vi "Normalize.vi"(11 "Data":dbl[][](array[numeric])) -> (0 "sx_all":dbl[][](array[numeric]), 2 "sx":dbl[](array[numeric]), 3 "Data_out":dbl[][](array[numeric]))   [LabVIEW 2014]
uses:
  <vilib>/Analysis/NI_AALBase.lvlib
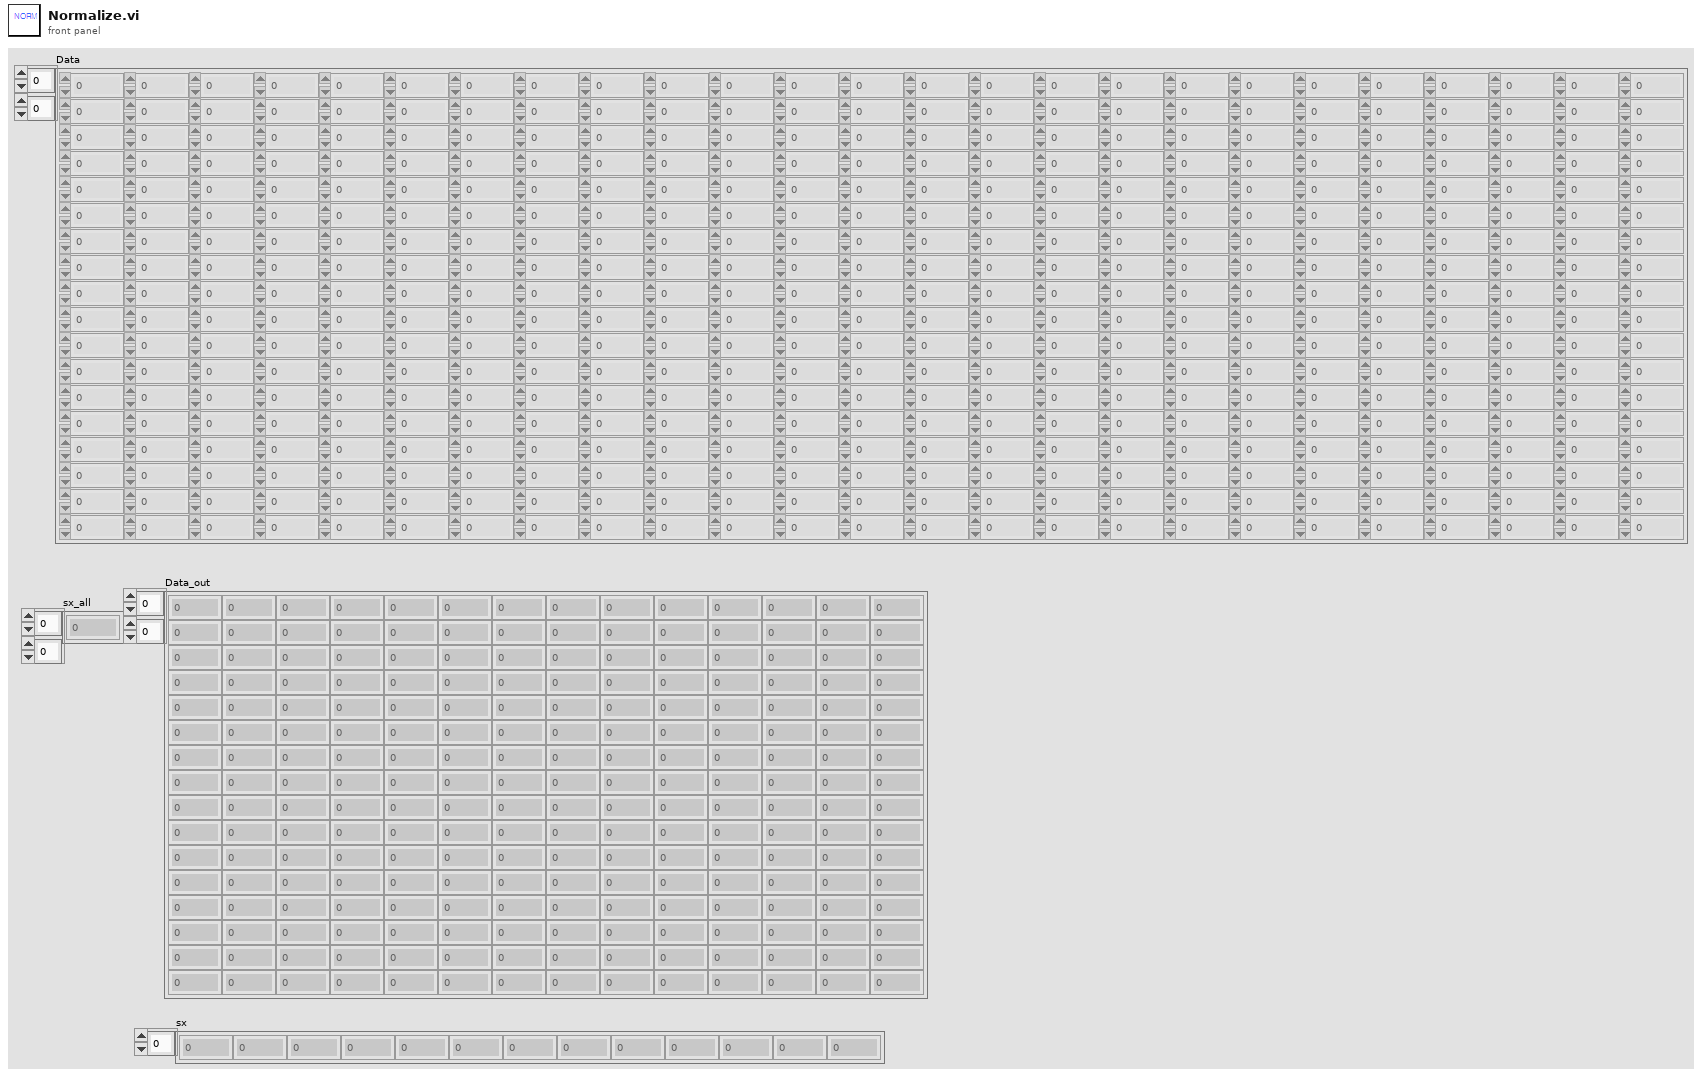
[diagram p1: front panel]
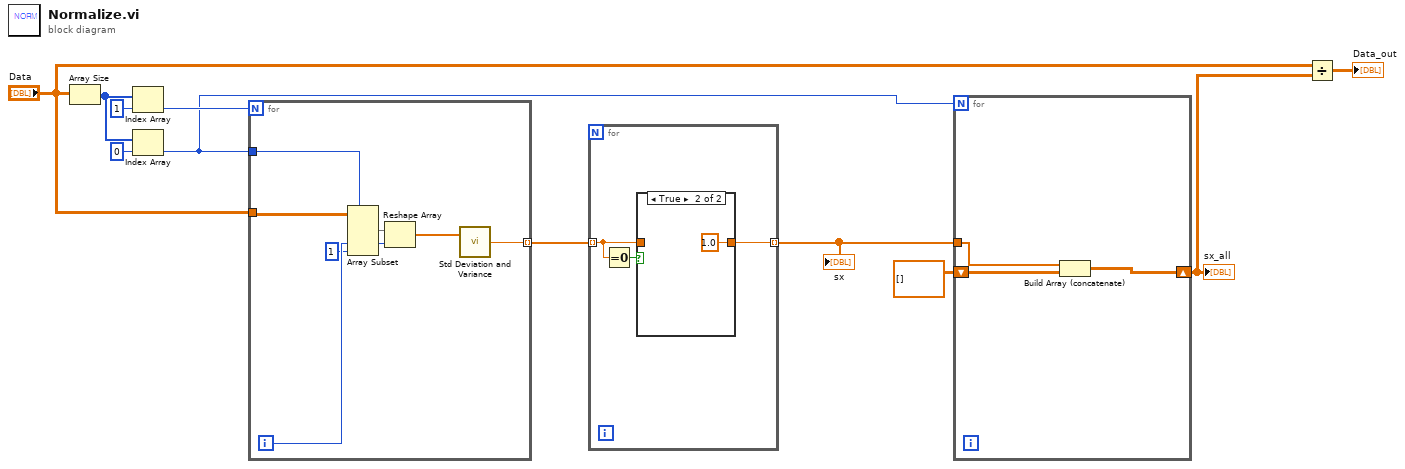
[diagram p0: block diagram]
diagram:
  n1 = Array Size(array="Data") -> (size(s)=w8:i32[])
  n2 = Index Array(array=w8, index=1) -> (element=w10:i32)
  n3 = Index Array(array=w8, index=0) -> (element=w7:i32)
  n4 = for {
    N: w10 -> [_]
    tunnel: "Data" -> [w18]
    tunnel: w7 -> [w14]
    tunnel: [w12] -> w2 mode=indexing
    i -> [w17]
    n5 = Array Subset(array=w18, index (col)=w17, length (col)=1 ("length")) -> (w15:dbl[][])  [unwired: 2 in]
    n6 = Reshape Array(w15, w14) -> (w13:dbl[])
    n7 = call <vilib>:"Std Deviation and Variance.vi"("X"=w13) -> ("standard deviation"=w12:dbl)  [unwired: 1 in, 2 out]
  }
  n8 = for {
    tunnel: w2 -> [w20] mode=indexing
    tunnel: [w19] -> w1 mode=indexing
    n9 = Equal To 0?(x=w20) -> (x = 0?=w21:bool)
    n10 = case shown="True" w21 {
      tunnel: w20 -> [w22 _]
      tunnel: [w22 1.0 ("standard deviation")] -> w19
      frame False {
      }
      frame True {
      }
    }
  }
  "sx" <- w1
  n11 = for {
    N: w7 -> [_]
    tunnel: w1 -> [w26]
    shift-right: [w25] -> w4
    shift-left: dbl[][] [] -> [w24]
    n12 = Build Array (concatenate)(w26, w24) -> (w25:dbl[][])
  }
  "sx_all" <- w4
  n13 = Divide(x="Data", y=w4) -> (x/y=→"Data_out":dbl[][])
